vi "Triggers To Buttons.vi"(11 "Axes":dbl[](array[numeric])) -> (2 "Right":bool, 3 "Left":bool)   [LabVIEW 2015]
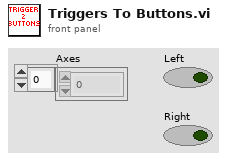
[diagram p1: front panel]
types:
  T1 = cluster{"Axes[0]":dbl, "Axes[1]":dbl, "Axes[2]":dbl, "Axes[3]":dbl, "Axes[4]":dbl, "Axes[5]":dbl, "Axes[6]":dbl, "Axes[7]":dbl, "Axes[8]":dbl}
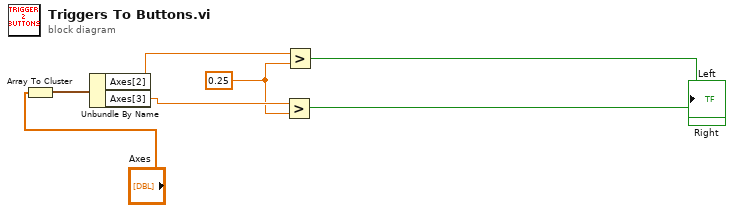
[diagram p0: block diagram]
diagram:
  w1 = 0.25 ("y")
  n1 = Array To Cluster(array="Axes") -> (cluster=w2:T1)
  n2 = Unbundle By Name(w2) -> ("Axes[2]"=w3:dbl, "Axes[3]"=w5:dbl)
  n3 = Greater?(x=w5, y=w1) -> (0:→"Right":bool)
  n4 = Greater?(x=w3, y=w1) -> (0:→"Left":bool)
